vi "Read Interrupt StatusHW.vi"(8 "error in (no error)":errorcluster, 11 "BME_DG_Base in":refnum<class "BME_DG_Base.lvclass">) -> (0 "error out":errorcluster, 2 "Interrupt Status":u32, 3 "BME_DG_Base out":refnum<class "BME_DG_Base.lvclass">)   [LabVIEW 2009, in "POLARIS BME DG.lvlib" / "BME_DG_Base.lvclass"]
uses:
  BME_DG_Base.lvclass
  BME_DG_Base.lvclass/BME_DG_Base.ctl
  POLARIS BME DG.lvlib
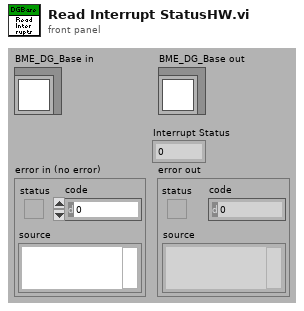
[diagram p1: front panel]
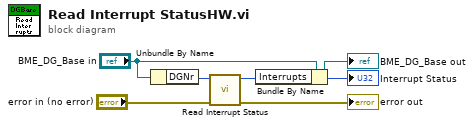
[diagram p0: block diagram]
diagram:
  n1 = Unbundle By Name("BME_DG_Base in") -> ("DGNr"=w5:i32)
  n2 = call "Read Interrupt Status.vi"("error in (no error)"="error in (no error)", "DG Number"=w5) -> ("error out"=→"error out":errorcluster, "Interrupt Status"=w1:u32)  [unwired: 8 in]
  "Interrupt Status" <- w1
  n3 = Bundle By Name(cluster="BME_DG_Base in", "Interrupts"=w1) -> (→"BME_DG_Base out":refnum<class "BME_DG_Base.lvclass">)
